vi "ConfigUpdateProgram.vi"(7 "MulticolumnListbox in":refnum<vi>, 8 "New Element":string[](array[string]), 10 "Operation":u16(ring)=1 items=["Append"=1, "Insert"=2, "Replace"=4], 11 "ItemNames in":string[][](array[string])) -> (3 "ItemNames out":string[][](array[string]))   [LabVIEW 2018, in "Config.lvlib"]
uses:
  Config.lvlib
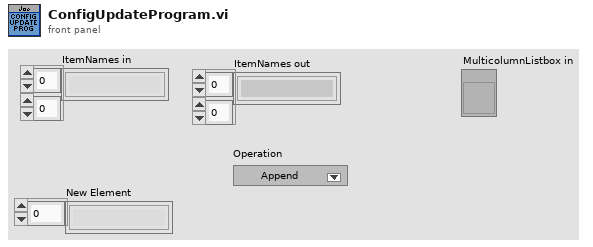
[diagram p1: front panel]
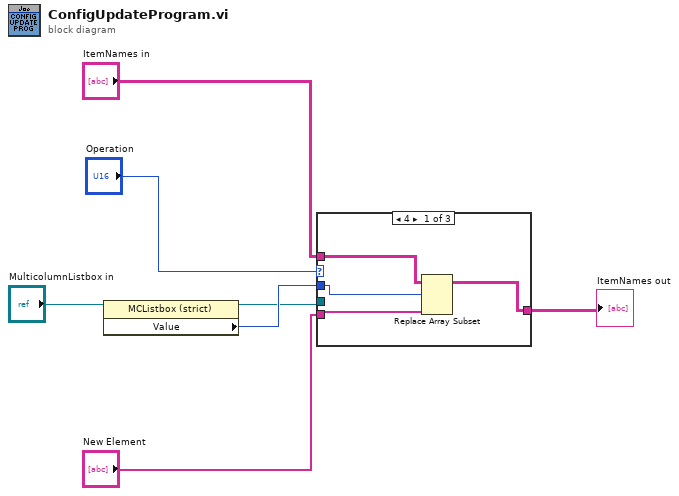
[diagram p0: block diagram]
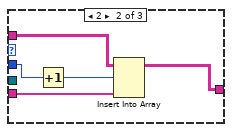
[diagram p2: hidden frame]
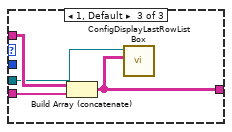
[diagram p3: hidden frame]
diagram:
  n1 = property class="MCListbox (strict)"(reference="MulticolumnListbox in") -> (reference out=w1:refnum<vi>, "Value"=w2:i32)  [unwired: 1 in, 1 out]
  n2 = case shown="4" "Operation" {
    tunnel: "New Element" -> [w10 w15 w20]
    tunnel: "ItemNames in" -> [w11 w16 w19]
    tunnel: [w9 w14 w18] -> w7
    tunnel: w1 -> [_ _ w17]
    tunnel: w2 -> [w8 w13 _]
    frame 4 {
      n3 = Replace Array Subset(array=w11, new element=w10, index (row)=w8) -> (w9:string[][])  [unwired: 1 in]
    }
    frame 2 {
      n4 = Increment(x=w13) -> (x+1=w12:i32)
      n5 = Insert Into Array(array=w16, index (row)=w12, new element=w15) -> (w14:string[][])  [unwired: 1 in]
    }
    frame 1, Default {
      n6 = Build Array (concatenate)(w19, w20) -> (w18:string[][])
      n7 = call "ConfigDisplayLastRowListBox.vi"("Array"=w18, "reference"=w17) -> ()  [unwired: 10 in]
    }
  }
  "ItemNames out" <- w7
